vi "Set Tag.vi"(7 "Persistant":bool, 8 "error in (no error)":errorcluster, 9 "Tag Value":string, 10 "TagName":string="phygbuTag", 11 "reference":refnum<vi>) -> (0 "error out":errorcluster, 2 "Old value":string, 3 "reference Out":refnum<vi>)   [LabVIEW 2012, in "Scripting Tools.lvlib"]
doc: "Sets a string tag on a LabVIEW object given by the reference input, optionally making the tag persistent. This is useful for later wiring."
uses:
  Scripting Tools.lvlib
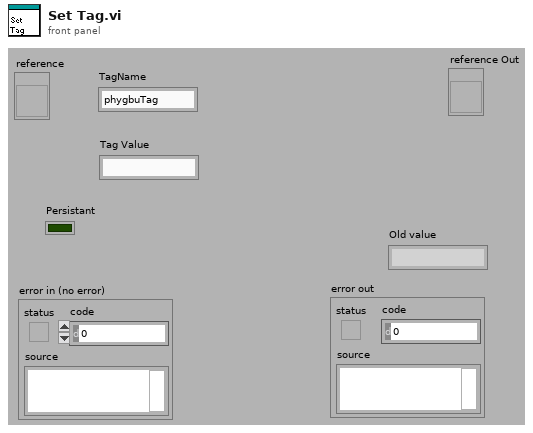
[diagram p1: front panel]
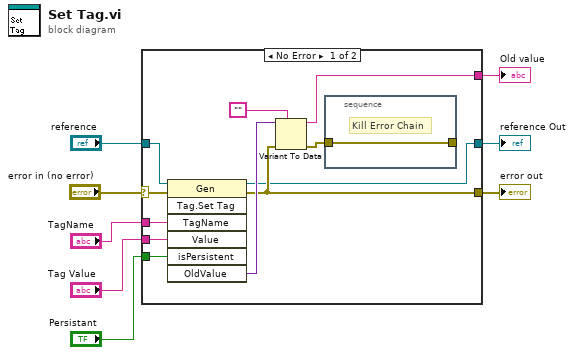
[diagram p0: block diagram]
diagram:
  n1 = case shown="No Error" "error in (no error)" {
    selector: "error in (no error)" -> [w18 w21]
    tunnel: "reference" -> [w19 w22]
    tunnel: "TagName" -> [w17 _]
    tunnel: "Tag Value" -> [w16 _]
    tunnel: "Persistant" -> [w15 _]
    tunnel: [w12 _] -> w3
    tunnel: [w11 w21] -> w2
    tunnel: [w10 w22] -> w1
    frame No Error {
      n2 = invoke on="Invoke Node" class="Gen" method="Tag.Set Tag"(reference=w19, error in=w18, "TagName"=w17, "Value"=w16, "isPersistent"=w15) -> (reference out=w10:refnum<vi>, error out=w11:errorcluster, "OldValue"=w14:variant)  [unwired: 2 in, 4 out]
      n3 = Variant To Data(error in=w11, type="" ("Empty String Constant"), Variant=w14) -> (data=w12:string, error out=w9:errorcluster)
      n4 = stacked-sequence {
        tunnel: [w20] -> _
        tunnel: w9 -> [w20]
        frame #0 {
          # "Kill Error Chain"
        }
      }
    }
    frame Error {
    }
  }
  "error out" <- w2
  "reference Out" <- w1
  "Old value" <- w3
